vi "AlazarErrorToText.vi"(1 "Message":string, 2 "Error Code":u32) -> (0 "Text":string)   [LabVIEW 2009]
doc: "Convert a numerical return code to a NULL terminated string."
uses:
  ATSApi.dll
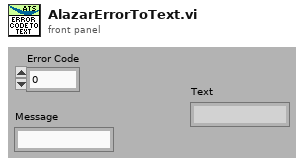
[diagram p1: front panel]
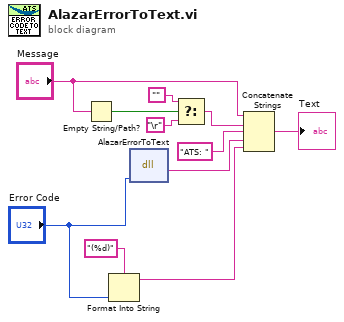
[diagram p0: block diagram]
diagram:
  n1 = Empty String/Path?(string/path="Message") -> (empty?=w3:bool)
  n2 = Format Into String(format string="(%d)", "Error Code") -> (resulting string=w7:string)  [unwired: 2 in, 1 out]
  n3 = dll-call lib="ATSApi.dll" fn="AlazarErrorToText"("ErrorCode"="Error Code") -> (w6:string)  [unwired: 4 in, 2 out]
  n4 = Select(t="", s=w3, f="\r") -> (s? t:f=w9:string)
  n5 = Concatenate Strings("Message", w9, "ATS: ", w6, w7) -> (→"Text":string)
